vi "OpenPhidget.vi"   [LabVIEW 2020]
uses:
  <instrlib>/Phidgets/Phidget Accelerometer/Phidget Accelerometer.lvlib
  <instrlib>/Phidgets/Phidget Current Input/Phidget Current Input.lvlib
  <instrlib>/Phidgets/Phidget DC Motor/Phidget DC Motor.lvlib
  <instrlib>/Phidgets/Phidget Digital Input/Phidget Digital Input.lvlib
  <instrlib>/Phidgets/Phidget Digital Output/Phidget Digital Output.lvlib
  <instrlib>/Phidgets/Phidget Encoder/Phidget Encoder.lvlib
  <instrlib>/Phidgets/Phidget Frequency Counter/Phidget Frequency Counter.lvlib
  <instrlib>/Phidgets/Phidget GPS/Phidget GPS.lvlib
  <instrlib>/Phidgets/Phidget Gyroscope/Phidget Gyroscope.lvlib
  <instrlib>/Phidgets/Phidget Humidity Sensor/Phidget Humidity Sensor.lvlib
  <instrlib>/Phidgets/Phidget IR/Phidget IR.lvlib
  <instrlib>/Phidgets/Phidget LCD/Phidget LCD.lvlib
  <instrlib>/Phidgets/Phidget Light Sensor/Phidget Light Sensor.lvlib
  <instrlib>/Phidgets/Phidget Magnetometer/Phidget Magnetometer.lvlib
  <instrlib>/Phidgets/Phidget Pressure Sensor/Phidget Pressure Sensor.lvlib
  <instrlib>/Phidgets/Phidget RC Servo/Phidget RC Servo.lvlib
  <instrlib>/Phidgets/Phidget RFID/Phidget RFID.lvlib
  <instrlib>/Phidgets/Phidget Spatial/Phidget Spatial.lvlib
  <instrlib>/Phidgets/Phidget Stepper/Phidget Stepper.lvlib
  <instrlib>/Phidgets/Phidget Temperature Sensor/Phidget Temperature Sensor.lvlib
  <instrlib>/Phidgets/Phidget Voltage Input/Phidget Voltage Input.lvlib
  <instrlib>/Phidgets/Phidget Voltage Output/Phidget Voltage Output.lvlib
  <instrlib>/Phidgets/Phidget Voltage Ratio Input/Phidget Voltage Ratio Input.lvlib
  <instrlib>/Phidgets/Phidget Capacitive Touch/Phidget Capacitive Touch.lvlib
  <instrlib>/Phidgets/Phidget PH Sensor/Phidget PH Sensor.lvlib
  <instrlib>/Phidgets/Phidget Distance Sensor/Phidget Distance Sensor.lvlib
  <instrlib>/Phidgets/Phidget Sound Sensor/Phidget Sound Sensor.lvlib
  <instrlib>/Phidgets/Phidget Resistance Input/Phidget Resistance Input.lvlib
  <instrlib>/Phidgets/Phidget Power Guard/Phidget Power Guard.lvlib
  <instrlib>/Phidgets/Phidget Motor Position Controller/Phidget Motor Position Controller.lvlib
  <instrlib>/Phidgets/Phidget BLDC Motor/Phidget BLDC Motor.lvlib
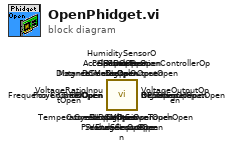
[diagram p0: block diagram]
diagram:
  n1 = call <instrlib>:"BLDCMotorOpen.vi"() -> ()  [unwired: 8 in, 4 out]
  n2 = call <instrlib>:"MotorPositionControllerOpen.vi"() -> ()  [unwired: 8 in, 4 out]
  n3 = call <instrlib>:"PowerGuardOpen.vi"() -> ()  [unwired: 8 in, 4 out]
  n4 = call <instrlib>:"ResistanceInputOpen.vi"() -> ()  [unwired: 8 in, 4 out]
  n5 = call <instrlib>:"SoundSensorOpen.vi"() -> ()  [unwired: 8 in, 4 out]
  n6 = call <instrlib>:"DistanceSensorOpen.vi"() -> ()  [unwired: 8 in, 4 out]
  n7 = call <instrlib>:"PHSensorOpen.vi"() -> ()  [unwired: 8 in, 4 out]
  n8 = call <instrlib>:"CapacitiveTouchOpen.vi"() -> ()  [unwired: 8 in, 4 out]
  n9 = call <instrlib>:"VoltageRatioInputOpen.vi"() -> ()  [unwired: 8 in, 4 out]
  n10 = call <instrlib>:"VoltageOutputOpen.vi"() -> ()  [unwired: 8 in, 4 out]
  n11 = call <instrlib>:"VoltageInputOpen.vi"() -> ()  [unwired: 8 in, 4 out]
  n12 = call <instrlib>:"TemperatureSensorOpen.vi"() -> ()  [unwired: 8 in, 4 out]
  n13 = call <instrlib>:"StepperOpen.vi"() -> ()  [unwired: 8 in, 4 out]
  n14 = call <instrlib>:"SpatialOpen.vi"() -> ()  [unwired: 8 in, 4 out]
  n15 = call <instrlib>:"RFIDOpen.vi"() -> ()  [unwired: 8 in, 4 out]
  n16 = call <instrlib>:"RCServoOpen.vi"() -> ()  [unwired: 8 in, 4 out]
  n17 = call <instrlib>:"PressureSensorOpen.vi"() -> ()  [unwired: 8 in, 4 out]
  n18 = call <instrlib>:"MagnetometerOpen.vi"() -> ()  [unwired: 8 in, 4 out]
  n19 = call <instrlib>:"LightSensorOpen.vi"() -> ()  [unwired: 8 in, 4 out]
  n20 = call <instrlib>:"LCDOpen.vi"() -> ()  [unwired: 8 in, 4 out]
  n21 = call <instrlib>:"IROpen.vi"() -> ()  [unwired: 8 in, 4 out]
  n22 = call <instrlib>:"HumiditySensorOpen.vi"() -> ()  [unwired: 8 in, 4 out]
  n23 = call <instrlib>:"GyroscopeOpen.vi"() -> ()  [unwired: 8 in, 4 out]
  n24 = call <instrlib>:"GPSOpen.vi"() -> ()  [unwired: 8 in, 4 out]
  n25 = call <instrlib>:"FrequencyCounterOpen.vi"() -> ()  [unwired: 8 in, 4 out]
  n26 = call <instrlib>:"EncoderOpen.vi"() -> ()  [unwired: 8 in, 4 out]
  n27 = call <instrlib>:"DigitalOutputOpen.vi"() -> ()  [unwired: 8 in, 4 out]
  n28 = call <instrlib>:"DigitalInputOpen.vi"() -> ()  [unwired: 8 in, 4 out]
  n29 = call <instrlib>:"DCMotorOpen.vi"() -> ()  [unwired: 8 in, 4 out]
  n30 = call <instrlib>:"CurrentInputOpen.vi"() -> ()  [unwired: 8 in, 4 out]
  n31 = call <instrlib>:"AccelerometerOpen.vi"() -> ()  [unwired: 8 in, 4 out]
